vi "resetView.vi"(8 "error in (no error)":errorcluster, 11 "CreditListUserInterface in":refnum<class "CreditListUAdapter.lvclass">) -> (0 "error out":errorcluster, 3 "CreditListUserInterface out":refnum<class "CreditListUAdapter.lvclass">)   [LabVIEW 2018, in "CreditListUAdapter.lvclass"]
uses:
  CreditListUAdapter.lvclass
  TransactionListUserInterface/TransactionListUIAdapter.lvclass
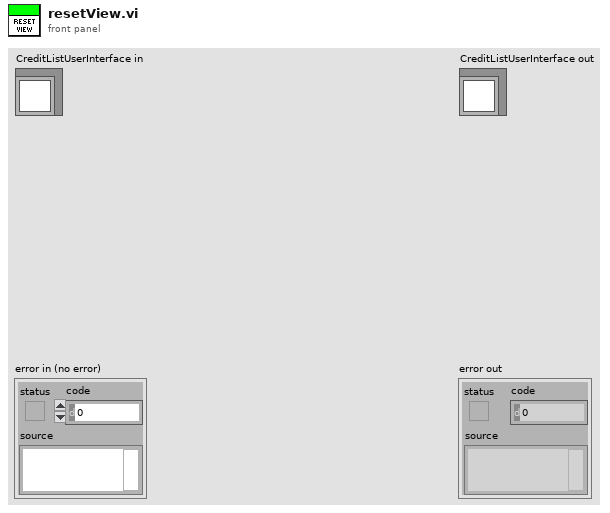
[diagram p1: front panel]
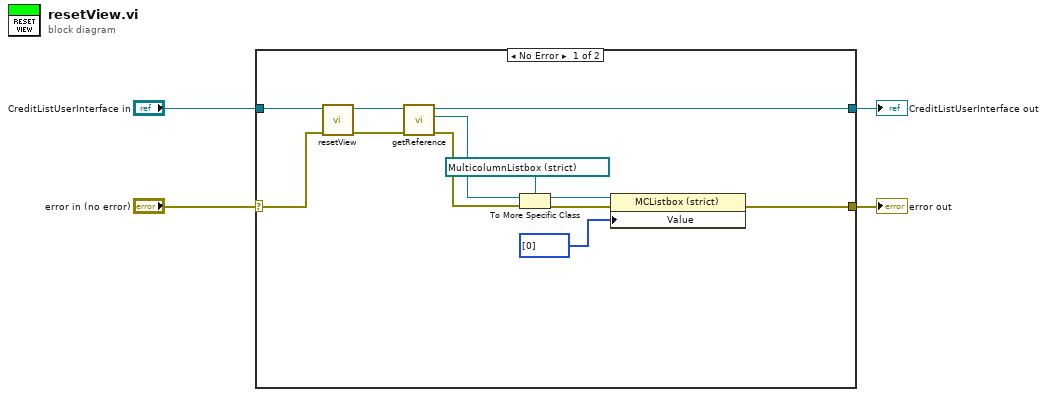
[diagram p0: block diagram]
diagram:
  n1 = case shown="No Error" "error in (no error)" {
    selector: "error in (no error)" -> [w14 w18]
    tunnel: [w16 w18] -> w3
    tunnel: [w11 w17] -> w1
    tunnel: "CreditListUserInterface in" -> [w15 w17]
    frame No Error {
      n2 = call-parent "resetView.vi"("error in (no error)"=w14, "TransactionListUserInterface in"=w15) -> ("error out"=w10:errorcluster, "TransactionListUserInterface out"=w12:refnum<class "CreditListUAdapter.lvclass">)  [unwired: 8 in]
      n3 = call-dynamic "getReference.vi"("error in (no error)"=w10, "TransactionListUserInterface in"=w12) -> ("error out"=w8:errorcluster, "MulticolumnListbox"=w9:refnum<vi>, "TransactionListUserInterface out"=w11:refnum<class "CreditListUAdapter.lvclass">)  [unwired: 7 in]
      n4 = To More Specific Class(target class=refnum<vi> refnum ("Credit"), reference=w9, error in=w8) -> (specific class reference=w6:refnum<vi>, error out=w7:errorcluster)
      n5 = property on="Property Node" class="MCListbox (strict)"(reference=w6, error in=w7, "Value"=i32[] [0] ("Credit")) -> (error out=w16:errorcluster)  [unwired: 1 out]
    }
    frame Error {
    }
  }
  "error out" <- w3
  "CreditListUserInterface out" <- w1
